vi "Build Control List.vi"(8 "error in (no error)":errorcluster, 11 "Generic Refnum":refnum<vi>) -> (0 "error out":errorcluster, 3 "Controls[] list":refnum<vi>[](array[refnum]))   [LabVIEW 2023]
doc: "Takes an array of references to controls and recursively builds an array containing those controls and any sub-controls (e.g., controls contained in a cluster in the list); however, does not include the clusters themselves in the output array.\n\nThis can be used to build an array of references to all controls in a VI by passing in the list of all controls on the front panel; see <B>Sensible Tab Order.vi</B> for an example."
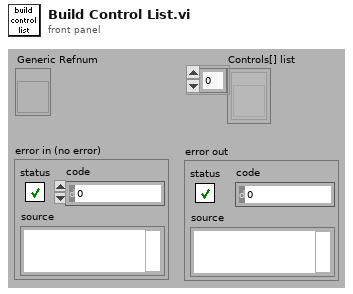
[diagram p1: front panel]
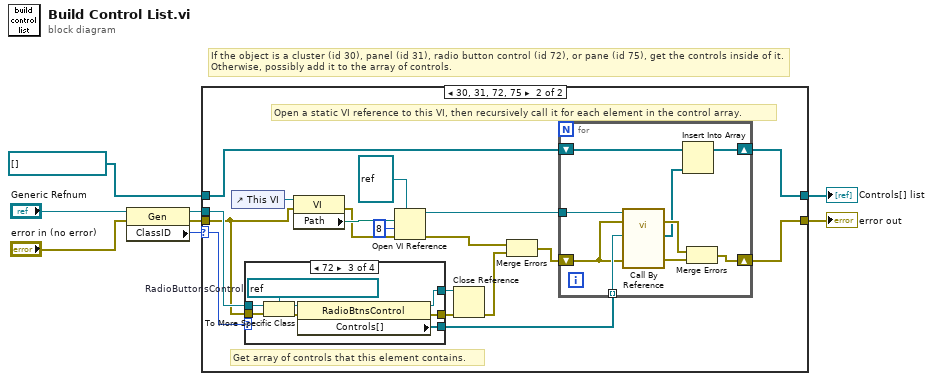
[diagram p0: block diagram]
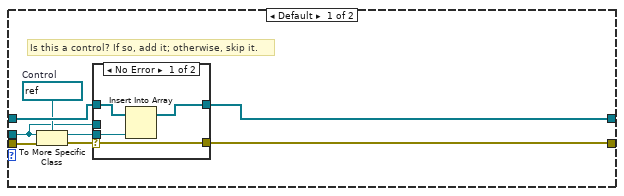
[diagram p2: hidden frame]
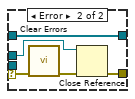
[diagram p3: hidden frame]
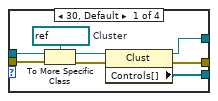
[diagram p4: hidden frame]
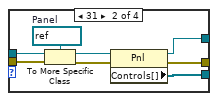
[diagram p5: hidden frame]
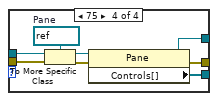
[diagram p6: hidden frame]
diagram:
  # "If the object is a cluster (id 30), panel (id 31), radio button control (id 72), or pane (id 75), get the controls inside of it. Otherwise, possibly add it to the array of controls."
  n1 = property class="Gen"(reference="Generic Refnum", error in="error in (no error)") -> (reference out=w3:refnum<vi>, error out=w2:errorcluster, "ClassID"=w4:u32)
  n2 = case shown="30, 31, 72, 75" w4 {
    selector: w4 -> [_ w35]
    tunnel: w3 -> [w9 w38]
    tunnel: w2 -> [w13 w33]
    tunnel: [w11 w36] -> w5
    tunnel: [w15 w30] -> w6
    tunnel: refnum<vi>[] [] ("Controls[]") -> [w16 w31]
    frame Default {
      w14 = refnum<vi> refnum  # Control
      # "Is this a control? If so, add it; otherwise, skip it."
      n3 = To More Specific Class(target class=w14, reference=w9, error in=w13) -> (specific class reference=w10:refnum<vi>, error out=w12:errorcluster)
      n4 = case shown="No Error" w12 {
        selector: w12 -> [w18 w25]
        tunnel: w16 -> [w20 w24]
        tunnel: [w19 w24] -> w15
        tunnel: [w18 w22] -> w11
        tunnel: w10 -> [w17 _]
        tunnel: w9 -> [_ w21]
        frame No Error {
          n5 = Insert Into Array(array=w20, new element=w17) -> (w19:refnum<vi>[])  [unwired: 1 in]
        }
        frame Error {
          n6 = call <vilib>:"Clear Errors.vi"("error in (no error)"=w25) -> ("error out"=w23:errorcluster)  [unwired: 1 in, 5 out]
          n7 = Close Reference(reference=w21, error in (no error)=w23) -> (error out=w22:errorcluster)
        }
      }
    }
    frame 30, 31, 72, 75 {
      # "Open a static VI reference to this VI, then recursively call it for each element in the control array."
      # "Get array of controls that this element contains."
      n8 = control-ref of="This VI"() -> (w39:refnum<vi>)
      n9 = case shown="72" w35 {
        tunnel: w38 -> [w60 w68 w76 w84]
        tunnel: [w57 w65 w73 w81] -> w37
        tunnel: w33 -> [w56 w64 w71 w80]
        tunnel: [w54 w62 w70 w78] -> w28
        tunnel: [w53 w61 w69 w77] -> w27
        frame 30, Default {
          w59 = refnum<vi> refnum  # Cluster
          n10 = To More Specific Class(target class=w59, reference=w60, error in=w56) -> (specific class reference=w58:refnum<vi>, error out=w55:errorcluster)
          n11 = property class="Clust"(reference=w58, error in=w55) -> (reference out=w53:refnum<vi>, error out=w54:errorcluster, "Controls[]"=w57:refnum<vi>[])
        }
        frame 31 {
          w67 = refnum<vi> refnum  # Panel
          n12 = To More Specific Class(target class=w67, reference=w68, error in=w64) -> (specific class reference=w66:refnum<vi>, error out=w63:errorcluster)
          n13 = property class="Pnl"(reference=w66, error in=w63) -> (reference out=w61:refnum<vi>, error out=w62:errorcluster, "Controls[]"=w65:refnum<vi>[])
        }
        frame 72 {
          w75 = refnum<vi> refnum  # RadioButtonsControl
          n14 = To More Specific Class(target class=w75, reference=w76, error in=w71) -> (specific class reference=w74:refnum<vi>, error out=w72:errorcluster)
          n15 = property class="RadioBtnsControl"(reference=w74, error in=w72) -> (reference out=w69:refnum<vi>, error out=w70:errorcluster, "Controls[]"=w73:refnum<vi>[])
        }
        frame 75 {
          w83 = refnum<vi> refnum  # Pane
          n16 = To More Specific Class(target class=w83, reference=w84, error in=w80) -> (specific class reference=w82:refnum<vi>, error out=w79:errorcluster)
          n17 = property class="Pane"(reference=w82, error in=w79) -> (reference out=w77:refnum<vi>, error out=w78:errorcluster, "Controls[]"=w81:refnum<vi>[])
        }
      }
      n18 = property class="VI"(reference=w39, error in=w33) -> (error out=w34:errorcluster, "Path"=w40:path)  [unwired: 1 out]
      n19 = Open VI Reference(type specifier VI Refnum (for type only)=refnum<vi> refnum, vi path=w40, options=8, error in (no error)=w34) -> (vi reference=w43:refnum<vi>, error out=w32:errorcluster)  [unwired: 2 out]
      n20 = Close Reference(reference=w27, error in (no error)=w28) -> (error out=w26:errorcluster)
      n21 = Merge Errors(w32, w26) -> (w29:errorcluster)
      n22 = for {
        tunnel: w43 -> [w50]
        tunnel: w37 -> [w49] mode=indexing
        shift-right: [w46] -> w30
        shift-left: w31 -> [w47]
        shift-right: [w48] -> w36
        shift-left: w29 -> [w44]
        n23 = call-by-ref "?"(reference=w50, error in=w44, 8:"error in (no error)"=w44, "Generic Refnum"=w49) -> (error out=w51:errorcluster, 0:"error out"=w52:errorcluster, "Controls[] list"=w45:refnum<vi>[])  [unwired: 8 in, 1 out]
        n24 = Insert Into Array(array=w47, new element=w45) -> (w46:refnum<vi>[])  [unwired: 1 in]
        n25 = Merge Errors(w51, w52) -> (w48:errorcluster)
      }
    }
  }
  "error out" <- w5
  "Controls[] list" <- w6
